vi "Fixture Input Monitor.vi"() -> ()   [LabVIEW 2010]
uses:
  <vilib>/DAQmx/read.llb/DAQmx Read (Digital U8 1Chan 1Samp).vi
  <vilib>/DAQmx/create/channels.llb/DAQmx Create Channel (DI-Digital Input).vi
  <vilib>/daqmx/miscellaneous.llb/DAQmx Fill In Error Info.vi
panel:
  out "Output Waiting For Reset":bool
  out "Doors Unlocked":bool
  in  "stop":bool
  out "I/O Fault":bool
  out "System Waiting for Reset":bool
  out "Bypass ON":bool
  out "Thermal Interlock OK":bool
  out "Crash Sensor OK":bool
  out "Rear Doors Closed":bool
  out "Front Right Door Closed":bool
  out "Front Left Doors Closed":bool
  out "E-Stops OK":bool
  out "Heat Zone 3 Flow B":bool
  out "Heat Zone 3 Flow A":bool
  # "The function of these inputs depends on how they are set-up in the flow sensor.\n Limit alarm, window or pulse train are possible."
  # "No E-stop is Pressed"
  # "\"Operator\" doors are closed but not necessarily locked."
  # "Front right door is closed but not necessarily locked"
  # "Rear doors are closed but not necessarily locked."
  # "3-Axis Motion Crash Sensor is not crashed."
  # "Thermostat on ceiling of chamber will open if it sees >50C"
  # "Guard doors are Bypassed. Motion will be enabled. State will cancel after set time."
  # "System Fault has occured. Must be manually reset. If it persists, see safety controller and it's documentation"
  # "A signal uncompatible with programmed safety input has been detected."
  # "System must lock the doors before safety circuit will be satisfied. Signal is negative logic."
  # "E-Stop or Crash Sensor tripped- Must be manually reset."
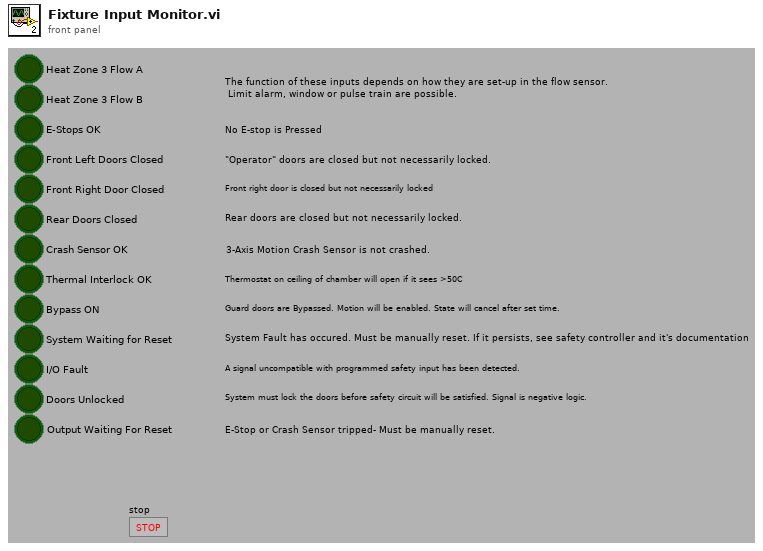
[diagram p1: front panel]
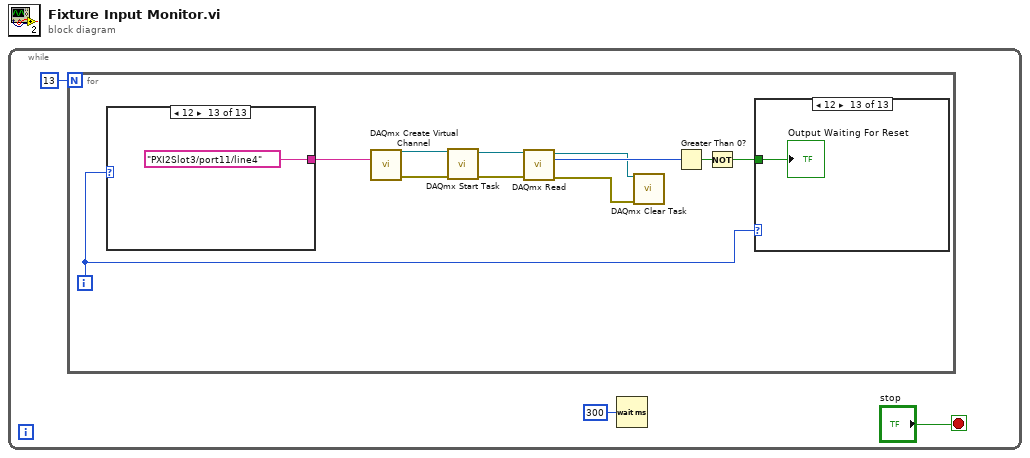
[diagram p0: block diagram]
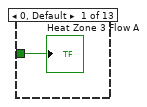
[diagram p2: hidden frame]
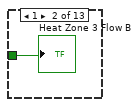
[diagram p3: hidden frame]
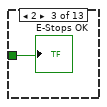
[diagram p4: hidden frame]
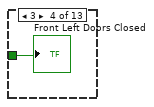
[diagram p5: hidden frame]
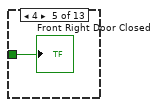
[diagram p6: hidden frame]
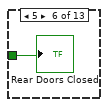
[diagram p7: hidden frame]
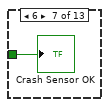
[diagram p8: hidden frame]
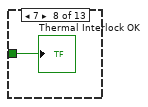
[diagram p9: hidden frame]
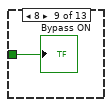
[diagram p10: hidden frame]
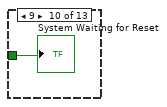
[diagram p11: hidden frame]
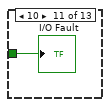
[diagram p12: hidden frame]
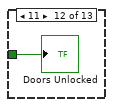
[diagram p13: hidden frame]
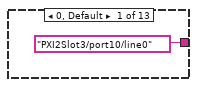
[diagram p14: hidden frame]
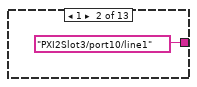
[diagram p15: hidden frame]
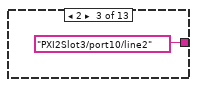
[diagram p16: hidden frame]
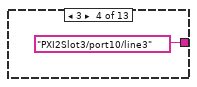
[diagram p17: hidden frame]
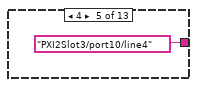
[diagram p18: hidden frame]
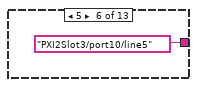
[diagram p19: hidden frame]
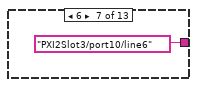
[diagram p20: hidden frame]
diagram:
  n1 = while {
    stop <- "stop" stop-if-true
    n2 = for {
      N: 13 -> [_]
      i -> [w9]
      n3 = case shown="12" w9 {
        tunnel: [tag "PXI2Slot3/port10/line0" ("Lines") tag "PXI2Slot3/port10/line1" ("Lines") tag "PXI2Slot3/port10/line2" ("Lines") tag "PXI2Slot3/port10/line3" ("Lines") tag "PXI2Slot3/port10/line4" ("Lines") tag "PXI2Slot3/port10/line5" ("Lines") tag "PXI2Slot3/port10/line6" ("Lines") tag "PXI2Slot3/port10/line7" ("Lines") tag "PXI2Slot3/port11/line0" ("Lines") tag "PXI2Slot3/port11/line1" ("Lines") tag "PXI2Slot3/port11/line2" ("Lines") tag "PXI2Slot3/port11/line3" ("Lines") tag "PXI2Slot3/port11/line4" ("Lines")] -> w14
        frame 0, Default {
        }
        frame 1 {
        }
        frame 2 {
        }
        frame 3 {
        }
        frame 4 {
        }
        frame 5 {
        }
        frame 6 {
        }
        frame 7 {
        }
        frame 8 {
        }
        frame 9 {
        }
        frame 10 {
        }
        frame 11 {
        }
        frame 12 {
        }
      }
      n4 = call-poly <vilib>:"DAQmx Create Virtual Channel.vi"("lines"=w14) -> ("task out"=w13:refnum<k21>, "error out"=w12:errorcluster)  [unwired: 13 in]
      n5 = call <vilib>:"DAQmx Start Task.vi"("task/channels in"=w13, "error in"=w12) -> ("task out"=w10:refnum<k21>, "error out"=w11:errorcluster)  [unwired: 12 in]
      n6 = call-poly <vilib>:"DAQmx Read.vi"("task/channels in"=w10, "error in"=w11) -> ("task out"=w6:refnum<k21>, "data"=w8:u8, "error out"=w5:errorcluster)  [unwired: 11 in]
      n7 = call <vilib>:"DAQmx Clear Task.vi"("task in"=w6, "error in"=w5) -> ()  [unwired: 13 in, 1 out]
      n8 = Greater Than 0?(x=w8) -> (x > 0?=w7:bool)
      n9 = Not(x=w7) -> (.not. x?=w4:bool)
      n10 = case shown="12" w9 {
        tunnel: w4 -> [w15 w16 w17 w18 w19 w20 w21 w22 w23 w24 w25 w26 w27]
        frame 0, Default {
          "Heat Zone 3 Flow A" <- w15
        }
        frame 1 {
          "Heat Zone 3 Flow B" <- w16
        }
        frame 2 {
          "E-Stops OK" <- w17
        }
        frame 3 {
          "Front Left Doors Closed" <- w18
        }
        frame 4 {
          "Front Right Door Closed" <- w19
        }
        frame 5 {
          "Rear Doors Closed" <- w20
        }
        frame 6 {
          "Crash Sensor OK" <- w21
        }
        frame 7 {
          "Thermal Interlock OK" <- w22
        }
        frame 8 {
          "Bypass ON" <- w23
        }
        frame 9 {
          "System Waiting for Reset" <- w24
        }
        frame 10 {
          "I/O Fault" <- w25
        }
        frame 11 {
          "Doors Unlocked" <- w26
        }
        frame 12 {
          "Output Waiting For Reset" <- w27
        }
      }
    }
    n11 = Wait (ms)(milliseconds to wait=u32 300) -> ()  [unwired: 1 out]
  }
